vi "SPI Engine Core 64-bit.vi"(6 "Ready for Output":bool, 9 "Input Valid":bool, 10 "SPI Transaction Packet":T1 {"SPI Settings"."SPI Physical Settings"."Direction Change Bit" max=64 step=1; "SPI Settings"."SPI Physical Settings"."Transfer Length (bits)" min=1 max=64 step=1}, 11 "SPI DIO Input":T7) -> (1 "Output Valid":bool, 2 "SPI Output Data":T5, 3 "SPI DIO Output":T6, 4 "Ready For Input":bool, 5 "Chip Select ID":u8)   [LabVIEW 2015, in "SPI API.lvlib"]
doc: "This VI performs the actual SPI Transactions. It wraps the SPI Core with added functionality of 4-Wire Handshake"
uses:
  SPI API.lvlib
  <userlib>/_NI SPI IP/FPGA/Controllers/Public/Spi Master Inputs.ctl
  <userlib>/_NI SPI IP/FPGA/Controllers/Public/Spi Master Outputs.ctl
  Controls/SPI API Response Data 64-bit.ctl
  Controls/SPI API Data 64-bit.ctl
  Controls/SPI API Transaction Packet 64-bit.ctl
  Controls/SPI Transaction Settings.ctl
  <userlib>/_NI SPI IP/FPGA/Controllers/Public/Transfer Settings.ctl
  SPI Engine.Core.Input Buffer 64-bit.vi
  Custom SPI IP/Spi Master 64-bit.vi
  SPI Engine.Core.Output Buffer 64-bit.vi
  <userlib>/_NI SPI IP/FPGA/Controllers/NI SPI IP FPGA.lvlib
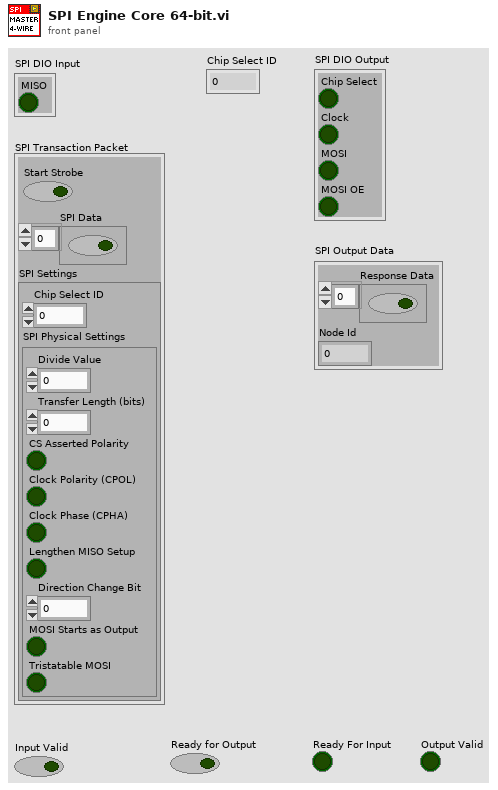
[diagram p1: front panel]
types:
  T1 = typedef "SPI API.lvlib/SPI API Transaction Packet 64-bit.ctl" = cluster{"Start Strobe":bool, "SPI Data":T2, "SPI Settings":T3}
  T2 = typedef "SPI API.lvlib/SPI API Data 64-bit.ctl" = bool[]
  T3 = typedef "SPI API.lvlib/SPI Transaction Settings.ctl" = cluster{"Chip Select ID":u8, "SPI Physical Settings":T4}
  T4 = typedef "NI SPI IP FPGA.lvlib/Transfer Settings.ctl" = cluster{"Divide Value":u8, "Transfer Length (bits)":u8, "CS Asserted Polarity":bool, "Clock Polarity (CPOL)":bool, "Clock Phase (CPHA)":bool, "Lengthen MISO Setup":bool, "Direction Change Bit":u8, "MOSI Starts as Output":bool, "Tristatable MOSI":bool}
  T5 = typedef "SPI API.lvlib/SPI API Response Data 64-bit.ctl" = cluster{"Response Data":T2, "Node Id":u16}
  T6 = typedef "NI SPI IP FPGA.lvlib/Spi Master Outputs.ctl" = cluster{"Chip Select":bool, "Clock":bool, "MOSI":bool, "MOSI OE":bool}
  T7 = typedef "NI SPI IP FPGA.lvlib/Spi Master Inputs.ctl" = cluster{"MISO":bool}
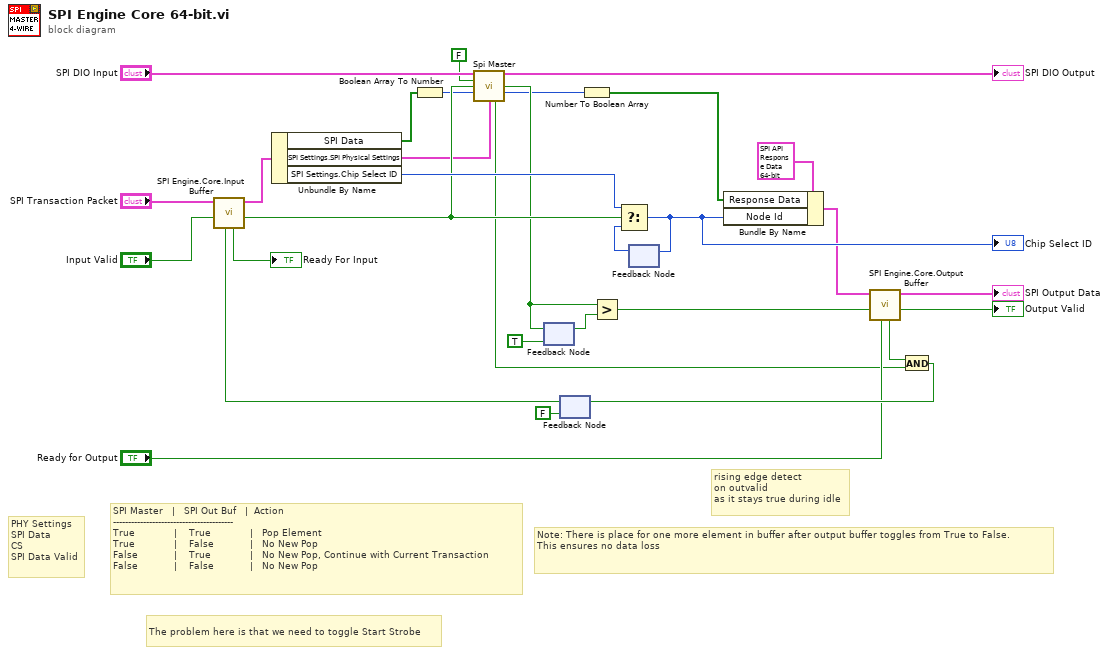
[diagram p0: block diagram]
diagram:
  # "rising edge detect\non outvalid\nas it stays true during idle"
  # "PHY Settings\nSPI Data\nCS\nSPI Data Valid"
  # "The problem here is that we need to toggle Start Strobe"
  # "Note: There is place for one more element in buffer after output buffer toggles from True to False.\nThis ensures no data loss"
  # "SPI Master   |   SPI Out Buf   |  Action\n----------------------------------------\nTrue             |    True             |   Pop Element\nTrue             |    False            |   No New Pop \nFalse            |    True             |   No New Pop, Continue with Current Transaction\nFalse            |    False            |   No New Pop"
  n1 = feedback #1(TRUE ("read data valid")) -> (w25:bool)
  n2 = feedback #2(FALSE) -> (w21:bool)
  n3 = call-poly "SPI Engine.Core.Input Buffer.vi"("Ready for Output"=w21, "Input Valid"="Input Valid", "SPI Information In"="SPI Transaction Packet") -> ("Output Valid"=w10:bool, "SPI Information Out"=w12:T1, "Ready For Input"=→"Ready For Input":bool)  [unwired: 6 in]
  n4 = Unbundle By Name(w12) -> ("SPI Data"=w1:T2, "SPI Settings.SPI Physical Settings"=w9:T4, "SPI Settings.Chip Select ID"=w23:u8)
  n5 = Boolean Array To Number(Boolean array=w1) -> (number=w2:u64)
  n6 = call-poly "Spi Master.vi"("spi input"="SPI DIO Input", "manual assert chip select"=FALSE, "start strobe"=w10, "data to write"=w2, "spi transfer settings"=w9) -> ("spi output"=→"SPI DIO Output":T6, "read data valid"=w6:bool, "read data"=w4:u64, "ready for input"=w8:bool)  [unwired: 7 in]
  n7 = feedback-in #1(w6) -> ()
  n8 = Number To Boolean Array(number=w4) -> (Boolean array=w3:bool[])
  n9 = Greater?(x=w6, y=w25) -> (0:w17:bool)
  n10 = feedback #3() -> (w27:u8)  [unwired: 1 in]
  n11 = Select(t=w23, s=w10, f=w27) -> (s? t:f=w24:u8)
  "Chip Select ID" <- w24
  n12 = feedback-in #3(w24) -> ()
  n13 = Bundle By Name(cluster=T5 {"Response Data"=[FALSE, FALSE, FALSE, FALSE, FALSE, FALSE, FALSE, FALSE, FALSE, FALSE, FALSE, FALSE, FALSE, FALSE, FALSE, FALSE, FALSE, FALSE, FALSE, FALSE, FALSE, FALSE, FALSE, FALSE, FALSE, FALSE, FALSE, FALSE, FALSE, FALSE, FALSE, FALSE, FALSE, FALSE, FALSE, FALSE, FALSE, FALSE, FALSE, FALSE, FALSE, FALSE, FALSE, FALSE, FALSE, FALSE, FALSE, FALSE, FALSE, FALSE, FALSE, FALSE, FALSE, FALSE, FALSE, FALSE, FALSE, FALSE, FALSE, FALSE, FALSE, FALSE, FALSE, FALSE], "Node Id"=0} ("SPI Response"), "Response Data"=w3, "Node Id"=w24) -> (w19:T5)
  n14 = call-poly "SPI Engine.Core.Output Buffer.vi"("Ready for Output"="Ready for Output", "Input Valid"=w17, "Input Data"=w19) -> ("Output Valid"=→"Output Valid":bool, "Output Data"=→"SPI Output Data":T5, "Ready For Input"=w14:bool)  [unwired: 6 in]
  n15 = And(x=w14, y=w8) -> (x .and. y?=w30:bool)
  n16 = feedback-in #2(w30) -> ()
